vi "ControlSolenoidValues (1).vi"() -> (3 "Solenoids Array":bool[](array[boolean]))   [LabVIEW 2017]
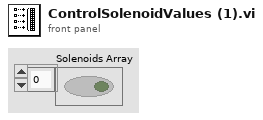
[diagram p1: front panel]
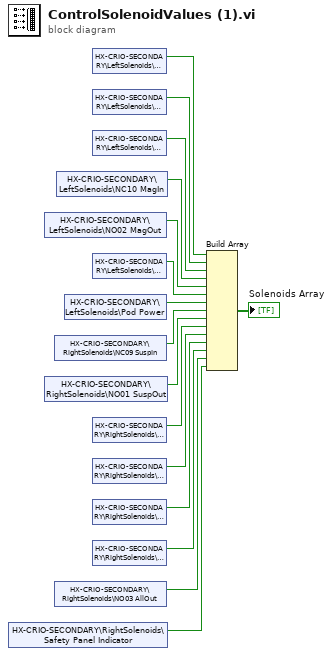
[diagram p0: block diagram]
diagram:
  n1 = shared-variable "HX-CRIO-SECONDARY\\RightSolenoids\\Safety Panel Indicator"() -> (w1:bool)  [unwired: 1 in, 1 out]
  n2 = shared-variable "HX-CRIO-SECONDARY\\LeftSolenoids\\NO02 MagOut"() -> (w11:bool)  [unwired: 1 in, 1 out]
  n3 = shared-variable "HX-CRIO-SECONDARY\\RightSolenoids\\NO01 SuspOut"() -> (w7:bool)  [unwired: 1 in, 1 out]
  n4 = shared-variable "HX-CRIO-SECONDARY\\RightSolenoids\\NC09 SuspIn"() -> (w8:bool)  [unwired: 1 in, 1 out]
  n5 = shared-variable "HX-CRIO-SECONDARY\\RightSolenoids\\NO03 AllOut"() -> (w2:bool)  [unwired: 1 in, 1 out]
  n6 = shared-variable "HX-CRIO-SECONDARY\\LeftSolenoids\\NC10 MagIn"() -> (w12:bool)  [unwired: 1 in, 1 out]
  n7 = shared-variable "HX-CRIO-SECONDARY\\LeftSolenoids\\Pod Power"() -> (w9:bool)  [unwired: 1 in, 1 out]
  n8 = shared-variable "HX-CRIO-SECONDARY\\LeftSolenoids\\NC03"() -> (w15:bool)  [unwired: 1 in, 1 out]
  n9 = shared-variable "HX-CRIO-SECONDARY\\LeftSolenoids\\NC04"() -> (w14:bool)  [unwired: 1 in, 1 out]
  n10 = shared-variable "HX-CRIO-SECONDARY\\LeftSolenoids\\NC02"() -> (w13:bool)  [unwired: 1 in, 1 out]
  n11 = shared-variable "HX-CRIO-SECONDARY\\LeftSolenoids\\NC01"() -> (w10:bool)  [unwired: 1 in, 1 out]
  n12 = shared-variable "HX-CRIO-SECONDARY\\RightSolenoids\\NC08"() -> (w6:bool)  [unwired: 1 in, 1 out]
  n13 = shared-variable "HX-CRIO-SECONDARY\\RightSolenoids\\NC05"() -> (w5:bool)  [unwired: 1 in, 1 out]
  n14 = shared-variable "HX-CRIO-SECONDARY\\RightSolenoids\\NC06"() -> (w4:bool)  [unwired: 1 in, 1 out]
  n15 = shared-variable "HX-CRIO-SECONDARY\\RightSolenoids\\NC07"() -> (w3:bool)  [unwired: 1 in, 1 out]
  n16 = Build Array(w15, w14, w13, w12, w11, w10, w9, w8, w7, w6, w5, w4, w3, w2, w1) -> (→"Solenoids Array":bool[])
